vi "Image Loader.vi"(3 "File Path":path=path "C:/Users/Mengchen/20120710/Sa02631.png") -> (1 "Last Scan Image":T1(plugin-control))   [LabVIEW 2013]
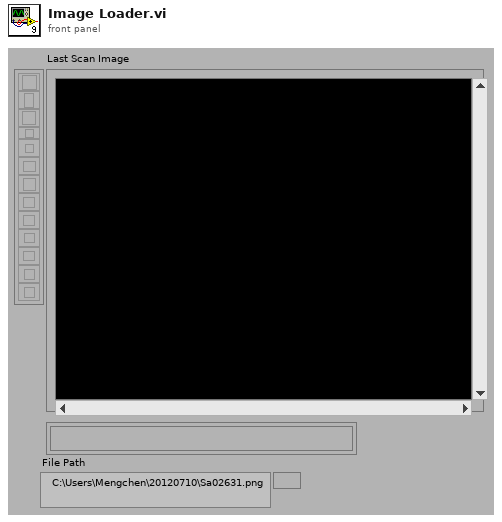
[diagram p1: front panel]
types:
  T1 = typedef "IMAQ Image.ctl" = refnum<image>
  T2 = typedef "Image Type" = u32
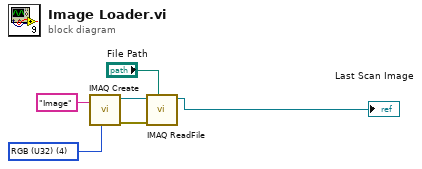
[diagram p0: block diagram]
diagram:
  w3 = T2 4 items=["Grayscale (U8)", "Grayscale (I16)", "Grayscale (SGL)", "Complex (CSG)", "RGB (U32)", "HSL (U32)", "RGB (U64)"] ("Image Type")
  n1 = call "IMAQ Create"("Image Name"="Image", "Image Type"=w3) -> ("New Image"=w5:T1, "error out"=w4:errorcluster)  [unwired: 2 in, 1 out]
  n2 = call "IMAQ ReadFile"("File Path"="File Path", "error in (no error)"=w4, "Image"=w5) -> ("Image Out"=→"Last Scan Image":T1)  [unwired: 2 in, 6 out]
